vi "Read Holding Registers1.vi"(7 "Unit_ID":T1={"Protocol ID"=0, "Unit ID"=1}, 8 "error in (no error)":errorcluster, 9 "number of holding registers":u16, 10 "starting address":u16, 11 "Modbus master in":refnum<class "TCP.lvclass">) -> (0 "error out":errorcluster, 2 "register values":u16[](array[numeric]), 3 "Modbus master out":refnum<class "TCP.lvclass">)   [LabVIEW 2019, in "NI_modbus_upd.lvlib"]
doc: "Reads values from contiguous holding registers. The maximum number of holding registers this VI can read is 125."
uses:
  NI_modbus_upd.lvlib
  TCP/TCP.lvclass
  Ctl/Unit_ID.ctl
  TCP/TCP.lvclass/TCP.ctl
  Utility/Bytes to U16s1.vi
  Function code mismatch error1.vi
  Error Generator1.vi
  Modbus Data Unit (PDU)/Construct PDU1.vi
  Read ADU Packet Master.vi
  Write ADU Packet Master.vi
  Modbus Data Unit (PDU)/Unflatten to PDU1.vi
  TCP/Protocol Read.vi
  TCP/Protocol Write.vi
  <vilib>/Utility/error.llb/Clear Errors.vi
  Modbus Data Unit (PDU)/Deconstruct PDU1.vi
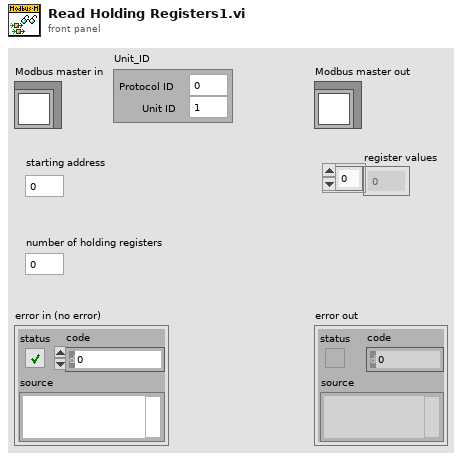
[diagram p1: front panel]
types:
  T1 = typedef "NI_modbus_upd.lvlib/Unit_ID.ctl" = cluster{"Protocol ID":u16, "Unit ID":u8}
  T2 = typedef "NI_modbus_upd.lvlib/MB Modbus Data Unit.ctl" = cluster{"function":T3, "Data":u8[]}
  T3 = typedef "NI_modbus_upd.lvlib/Function.ctl" = u8
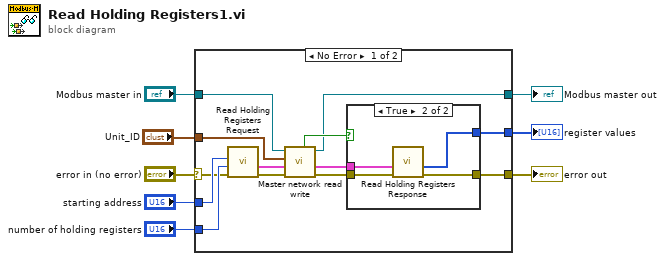
[diagram p0: block diagram]
diagram:
  n1 = case shown="No Error" "error in (no error)" {
    selector: "error in (no error)" -> [w13 w27]
    tunnel: "number of holding registers" -> [w17 _]
    tunnel: "starting address" -> [w18 _]
    tunnel: "Modbus master in" -> [w10 w28]
    tunnel: [w12 w28] -> w1
    tunnel: [w19 w27] -> w4
    tunnel: [w16 _] -> w3
    tunnel: "Unit_ID" -> [w9 _]
    frame No Error {
      n2 = call "Read Holding Registers Request.vi"("error in (no error)"=w13, "number of registers"=w17, "starting address"=w18) -> ("error out"=w20:errorcluster, "Modbus Data Unit out"=w14:T2)  [unwired: 7 in]
      n3 = call "Master network read write.vi"("error in (no error)"=w20, "Modbus Data Unit"=w14, "Unit_ID"=w9, "TCP in"=w10) -> ("error out"=w21:errorcluster, "Modbus data unit out"=w11:T2, "TCP out"=w12:refnum<class "TCP.lvclass">, "PDU valid?"=w15:bool)  [unwired: 4 in]
      n4 = case shown="True" w15 {
        tunnel: w21 -> [w22 w26]
        tunnel: [w22 w25] -> w19
        tunnel: [_ w24] -> w16
        tunnel: w11 -> [_ w23]
        frame False {
        }
        frame True {
          n5 = call "Read Holding Registers Response.vi"("error in (no error)"=w26, "Modbus Data Unit in"=w23) -> ("error out"=w25:errorcluster, "register values"=w24:u16[])  [unwired: 7 in, 1 out]
        }
      }
    }
    frame Error {
    }
  }
  "Modbus master out" <- w1
  "error out" <- w4
  "register values" <- w3
